vi "_mutatePropDef.vi"(10 "Object definitions":T4(array[cluster]), 11 "Selected properties":T1[](array[typedef])) -> (2 "Object definitions out":T5[](array[typedef]), 3 "Selected properties out":T1[](array[typedef]))   [LabVIEW 2017]
uses:
  <vilib>/Platform/storage/lvStorage.llb/dataModel.ctl
  <vilib>/Platform/storage/Storage.llb/usiTypeDef.ctl
  <vilib>/Platform/storage/Storage.llb/usiPropDef.ctl
  <vilib>/express/express shared/ex_EditUserDefinedProperties/usiDataType.ctl
  <vilib>/Platform/storage/Storage.llb/specialProperties.ctl
  <vilib>/Platform/storage/lvStorage.llb/_selectedProp.ctl
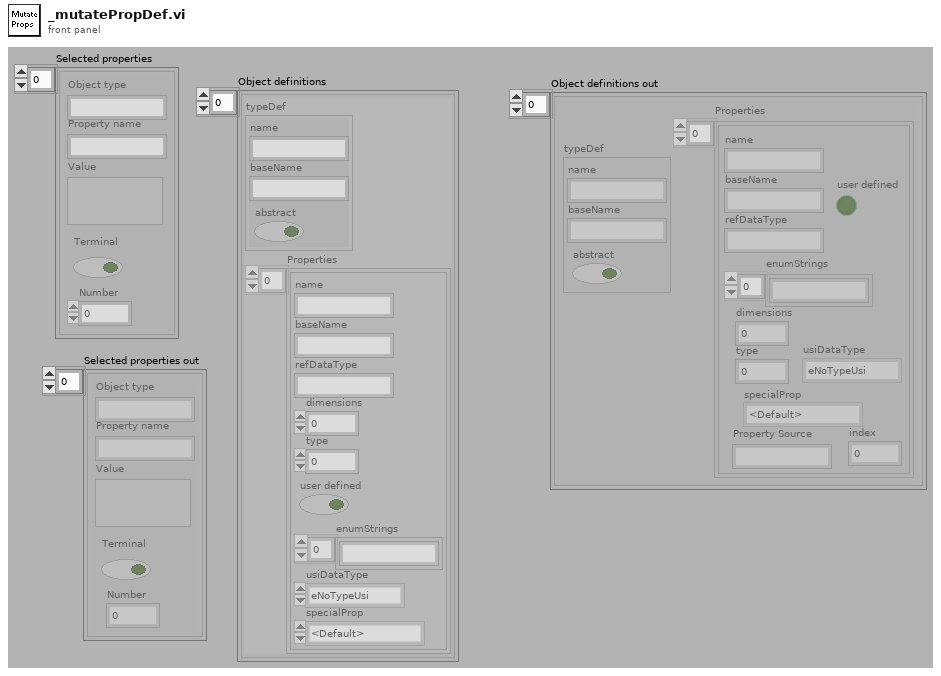
[diagram p1: front panel]
types:
  T1 = typedef "_selectedProp.ctl" = cluster{"Object type":string, "Property name":string, "Value":variant, "Terminal":bool, "Number":i32}
  T2 = typedef "usiTypeDef.ctl" = cluster{"name":string, "baseName":string, "abstract":bool}
  T3 = typedef "usiDataType.ctl" = enum16{"eNoTypeUsi", "eInt8Usi", "eInt16Usi", "eInt32Usi", "eInt64Usi", "eUInt8Usi", "eUInt16Usi", "eUInt32Usi", "eUInt64Usi", "eFloat32Usi", "eFloat64Usi", "- 0", "- 1", "- 2", "- 3", "- 4", "- 5", "- 6", "- 7", "- 8", "- 9", "eString8Usi", "eString16Usi", "eStringUsi", "eEnumUsi", "- 10", "- 11", "- 12", "- 13", "- 14", "eTimeUsi", "- 15", "- 16", "- 17", "- 18", "- 19", "- 20", "- 21", "- 22", "- 23", "eInstanceUsi", "eStoreUsi"}
  T4 = cluster{"typeDef":T2, "Properties":cluster{"name":string, "baseName":string, "refDataType":string, "dimensions":i32, "type":i32, "user defined":bool, "enumStrings":string[], "usiDataType":T3, "specialProp":enum16{"<Default>", "Channel Values", "AppendReplace", "ChannelFlags", "ValueFlags", "ImplicitExplicit", "InsertIndex", "ValuesCount", "ComparisonOperator", "Cluster"}}[]}[]
  T5 = typedef "dataModel.ctl" = cluster{"typeDef":T2, "Properties":T6[]}
  T6 = typedef "usiPropDef.ctl" = cluster{"name":string, "baseName":string, "refDataType":string, "dimensions":i32, "type":i32, "user defined":bool, "enumStrings":string[], "usiDataType":T3, "specialProp":T7, "Property Source":string, "index":i32}
  T7 = typedef "specialProperties.ctl" = enum16{"<Default>", "Channel Values", "AppendReplace", "ChannelFlags", "ValueFlags", "ImplicitExplicit", "InsertIndex", "ValuesCount", "ComparisonOperator", "Cluster", "DAQmx Channel"}
  T8 = cluster{"name":string, "baseName":string, "refDataType":string, "dimensions":i32, "type":i32, "user defined":bool, "enumStrings":string[], "usiDataType":T3, "specialProp":enum16{"<Default>", "Channel Values", "AppendReplace", "ChannelFlags", "ValueFlags", "ImplicitExplicit", "InsertIndex", "ValuesCount", "ComparisonOperator", "Cluster"}}[]
  T9 = enum16{"<Default>", "Channel Values", "AppendReplace", "ChannelFlags", "ValueFlags", "ImplicitExplicit", "InsertIndex", "ValuesCount", "ComparisonOperator", "Cluster"}
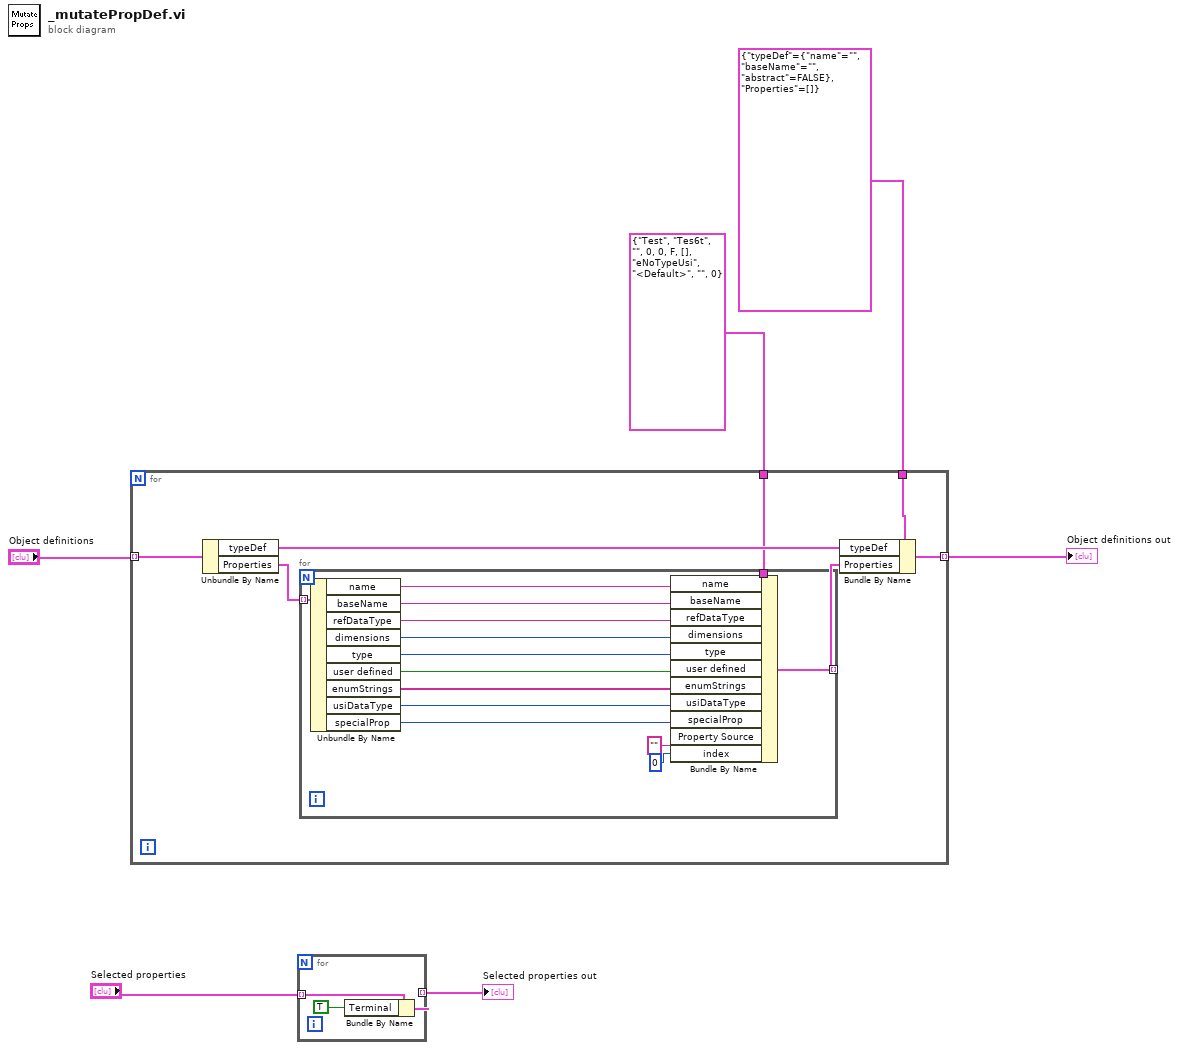
[diagram p0: block diagram]
diagram:
  n1 = for {
    tunnel: "Object definitions" -> [w13] mode=indexing
    tunnel: [w9] -> w6 mode=indexing
    tunnel: T6 {"name"="Test", "baseName"="Tes6t", "refDataType"="", "dimensions"=0, "type"=0, "user defined"=FALSE, "enumStrings"=[], "usiDataType"=enum."eNoTypeUsi", "specialProp"=enum."<Default>", "Property Source"="", "index"=0} ("propDef") -> [w10]
    tunnel: T5 {"typeDef"={"name"="", "baseName"="", "abstract"=FALSE}, "Properties"=[]} ("ObjectDefinition") -> [w7]
    n2 = Unbundle By Name(w13) -> ("typeDef"=w12:T2, "Properties"=w11:T8)
    n3 = for {
      tunnel: w11 -> [w26] mode=indexing
      tunnel: [w27] -> w8 mode=indexing
      tunnel: w10 -> [w25]
      n4 = Unbundle By Name(w26) -> ("name"=w24:string, "baseName"=w23:string, "refDataType"=w22:string, "dimensions"=w21:i32, "type"=w20:i32, "user defined"=w19:bool, "enumStrings"=w18:string[], "usiDataType"=w17:T3, "specialProp"=w14:T9)
      n5 = Bundle By Name(cluster=w25, "name"=w24, "baseName"=w23, "refDataType"=w22, "dimensions"=w21, "type"=w20, "user defined"=w19, "enumStrings"=w18, "usiDataType"=w17, "specialProp"=w14, "Property Source"="", "index"=0) -> (w27:T6)
    }
    n6 = Bundle By Name(cluster=w7, "typeDef"=w12, "Properties"=w8) -> (w9:T5)
  }
  "Object definitions out" <- w6
  n7 = for {
    tunnel: "Selected properties" -> [w30] mode=indexing
    tunnel: [w28] -> w1 mode=indexing
    n8 = Bundle By Name(cluster=w30, "Terminal"=TRUE) -> (w28:T1)
  }
  "Selected properties out" <- w1
